vi "DQMH Tester Prepare hse-appl - Get Name and Path.vi"(8 "error in":errorcluster, 11 "RT App Name or Path":string) -> (0 "error out":errorcluster, 2 "Project Path":path, 3 "Project Name":string)   [LabVIEW 2022 SP3, in "hse-dqmh.lvlib"]
doc: "Returns \nAPP-NAME as Project Name and \n/APP-NAME_Source as Project Path\n\nHSE projects follow this folder structure:\n /APP-NAME_Config .......... Configuration Files\n /APP-NAME_Data .............. Measured and Other Data\n /APP-NAME_Source .......... LabVIEW Sources\n /APP-NAME ........................ Compiled Application\n\nREAL-TIME: As the configuration directory on real-time systems always needs to reside at \"C:\\<Project Name>_Config\\\", and as it tedious (embedded UI) or impossible (no embedded UI) to enter the path, it can be supplied via the optional Real-Time App Name string input.\n\n____\nHAMPEL SOFTWARE ENGINEERING v3.8.0 (2023-12-18 14:41)"
uses:
  hse-dqmh.lvlib
  <vilib>/regexp/Match Regular Expression.xnode
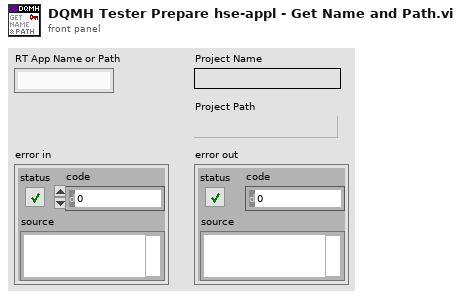
[diagram p1: front panel]
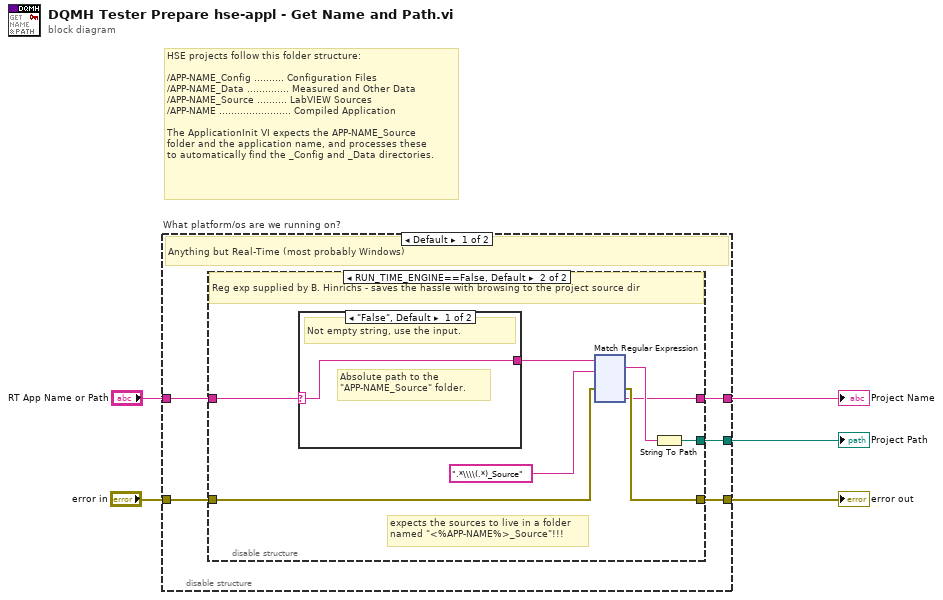
[diagram p0: block diagram]
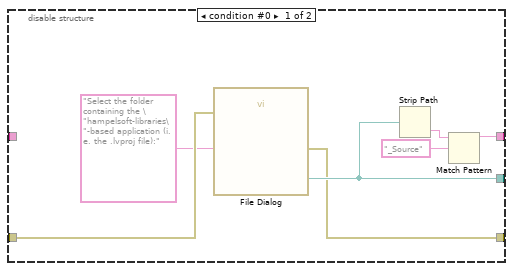
[diagram p2: hidden frame]
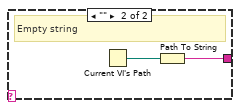
[diagram p3: hidden frame]
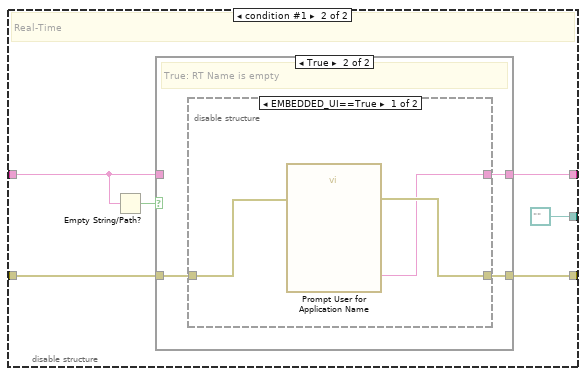
[diagram p4: hidden frame]
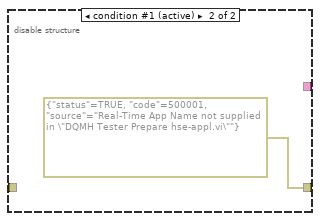
[diagram p6: hidden frame]
diagram:
  # "HSE projects follow this folder structure:\n\n/APP-NAME_Config .......... Configuration Files\n/APP-NAME_Data .............. Measured and Other Data\n/APP-NAME_Source .......... LabVIEW Sources\n/APP-NAME ........................ Compiled Application\n\nThe ApplicationInit VI expects the APP-NAME_Source\nfolder and the application name, and processes these\nto automatically find the _Config and _Data directories."
  n1 = disable-structure "What platform/os are we running on?" shown="Default" {
    disable-tunnel: [w10 path "" ("selected path")] -> w3
    disable-tunnel: [w9 w152] -> w4
    disable-tunnel: [w8 w153] -> w5
    disable-tunnel: "error in" -> [w7 w149]
    disable-tunnel: "RT App Name or Path" -> [w6 w148]
    frame condition #0 (active) {
      # "Anything but Real-Time (most probably Windows)"
      n2 = disable-structure shown="RUN_TIME_ENGINE==False, Default" {
        disable-tunnel: [w17 w20] -> w10
        disable-tunnel: [w14 w21] -> w9
        disable-tunnel: [w13 w25] -> w8
        disable-tunnel: w7 -> [w12 w19]
        disable-tunnel: w6 -> [_ w18]
        frame condition #0 {
          n3 = call "File Dialog"("prompt"="Select the folder containing the \"hampelsoft-libraries\"-based application (i.e. the .lvproj file):", "error in"=w12) -> ("selected path"=w17:path, "error out"=w13:errorcluster)  [unwired: 10 in, 2 out]
          n4 = Strip Path(path=w17) -> (name=w16:string)  [unwired: 1 out]
          n5 = Match Pattern(string=w16, regular expression="_Source") -> (before substring=w14:string)  [unwired: 1 in, 3 out]
        }
        frame condition #1 (active) {
          # "expects the sources to live in a folder \nnamed \"<%APP-NAME%>_Source\"!!!"
          # "Reg exp supplied by B. Hinrichs - saves the hassle with browsing to the project source dir"
          n6 = case shown="\"False\", Default" w18 {
            selector: w18 -> [w26 _]
            tunnel: [w26 w27] -> w24
            frame "False", Default {
              # "Absolute path to the\n\"APP-NAME_Source\" folder."
              # "Not empty string, use the input."
            }
            frame "" {
              # "Empty string"
              n7 = Current VI's Path() -> (path=w28:path)
              n8 = Path To String(path=w28) -> (string=w27:string)
            }
          }
          n9 = xnode "Match Regular Expression"("input string"=w24, "regular expression"=".*\\\\(.*)_Source", "error in"=w19) -> ("whole match"=w23:string, "error out"=w25:errorcluster, "submatch 1"=w21:string)  [unwired: 3 in, 3 out]
          n10 = String To Path(string=w23) -> (path=w20:path)
        }
      }
    }
    frame condition #1 {
      # "Real-Time"
      n11 = Empty String/Path?(string/path=w148) -> (empty?=w150:bool)
      n12 = case shown="True" w150 {
        tunnel: [w155 w158] -> w153
        tunnel: [w154 w157] -> w152
        tunnel: w149 -> [w155 w156]
        tunnel: w148 -> [w154 _]
        frame False {
          # "False: RT Name not empty"
        }
        frame True {
          # "True: RT Name is empty"
          n13 = disable-structure shown="EMBEDDED_UI==True" {
            disable-tunnel: [w161 errorcluster {"status"=TRUE, "code"=500001, "source"="Real-Time App Name not supplied in \"DQMH Tester Prepare hse-appl.vi\""} ("error out")] -> w158
            disable-tunnel: [w160 _] -> w157
            disable-tunnel: w156 -> [w159 _]
            frame condition #0 {
              n14 = call "Prompt User for Application Name"("error in (no error)"=w159) -> ("Application Name"=w160:string, "error out"=w161:errorcluster)  [unwired: 16 in, 1 out]
            }
            frame condition #1 (active) {
            }
          }
        }
      }
    }
  }
  "error out" <- w5
  "Project Name" <- w4
  "Project Path" <- w3
